vi "Write Address.vi"(8 "error in":errorcluster, 10 "Address":string, 11 "TCP master in":refnum<class "TCP Master.lvclass">) -> (0 "error out":errorcluster, 3 "TCP master out":refnum<class "TCP Master.lvclass">)   [LabVIEW 2013, in "Modbus Library - Advance.lvlib" / "TCP Master.lvclass"]
doc: "Property accessor for the TCP address."
uses:
  TCP Master.lvclass
  TCP Master.lvclass/TCP Master.ctl
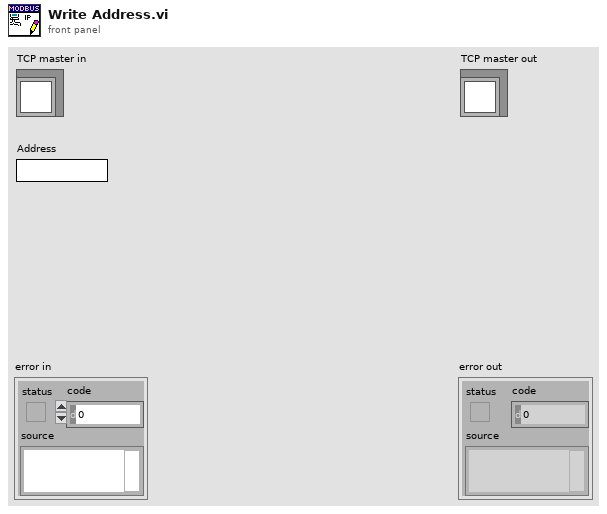
[diagram p1: front panel]
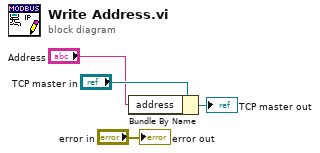
[diagram p0: block diagram]
diagram:
  n1 = Bundle By Name(cluster="TCP master in", "address"="Address") -> (→"TCP master out":refnum<class "TCP Master.lvclass">)
  "error out" <- "error in"
